vi "initialise.vi"(8 "error in (no error)":errorcluster, 11 "GenericPlugin in":refnum<class "StageMMS2015ASIfromScientifica.lvclass">) -> (0 "error out":errorcluster, 3 "GenericPlugin out":refnum<class "StageMMS2015ASIfromScientifica.lvclass">)   [LabVIEW 2010, in "StageMMS2015ASIfromScientifica.lvclass"]
doc: "The dynamic dispatch-version of this VI initalises the plug-in object by allocating and initalising any dynamic resources need."
uses:
  StageMMS2015ASIfromScientifica.lvclass
  StageDL090409Scaffold/StageDL090409Scaffold/StageDL090409Scaffold.lvclass
  <vilib>/Instr/_visa.llb/VISA Configure Serial Port (Instr).vi
  common/classes/ErrorController/ErrorController/class_data.vi
  common/classes/ErrorController/ErrorController/ErrorController.lvclass
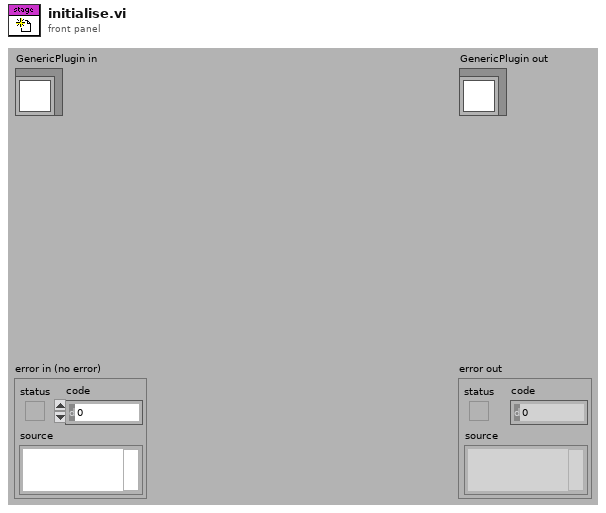
[diagram p1: front panel]
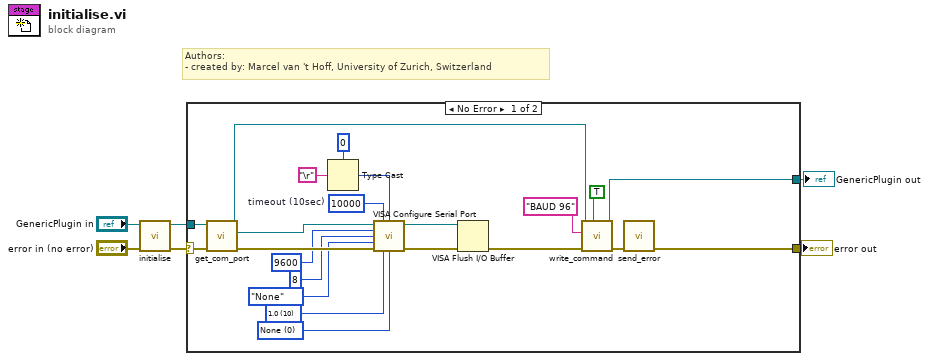
[diagram p0: block diagram]
diagram:
  # "Authors: \n- created by: Marcel van 't Hoff, University of Zurich, Switzerland"
  n1 = call-parent "initialise.vi"("error in (no error)"="error in (no error)", "GenericPlugin in"="GenericPlugin in") -> ("error out"=w4:errorcluster, "GenericPlugin out"=w1:refnum<class "StageMMS2015ASIfromScientifica.lvclass">)  [unwired: 8 in]
  n2 = case shown="No Error" w4 {
    selector: w4 -> [w26 w30]
    tunnel: [w14 w30] -> w3
    tunnel: [w17 w29] -> w2
    tunnel: w1 -> [w28 w29]
    frame No Error {
      w19 = u16 0 items=["None", "XON/XOFF", "RTS/CTS", "XON/XOFF & RTS/CTS", "DTR/DSR", "XON/XOFF & DTR/DSR"] ("flow control (0:none)")
      w20 = u16 10 items=["1.0"=10, "1.5"=15, "2.0"=20] ("stop bits (10: 1 bit)")
      w24 = u32 10000  # timeout (10sec)
      n3 = call-dynamic "get_com_port.vi"("error in (no error)"=w26, "StageMH110930Scientifica in"=w28) -> ("error out"=w25:errorcluster, "serial port name"=w27:refnum<visa-resource-name>, "StageMH110930Scientifica out"=w18:refnum<class "StageMMS2015ASIfromScientifica.lvclass">)  [unwired: 7 in]
      n4 = Type Cast(type=u8 0, x="\r") -> (*(type *) &x=w8:u8)
      n5 = call-poly "VISA Configure Serial Port"("VISA resource name"=w27, "timeout (10sec)"=w24, "termination char\n(0xA = '\\n' = LF)"=w8, "baud rate (9600)"=u32 9600, "data bits (8)"=u16 8, "parity (0:none)"=enum16{"None", "Odd", "Even", "Mark", "Space"}."None", "error in (no error)"=w25, "stop bits (10: 1 bit)"=w20, "flow control (0:none)"=w19) -> ("VISA resource name out"=w12:refnum<visa-resource-name>, "error out"=w11:errorcluster)  [unwired: 5 in]
      n6 = VISA Flush I/O Buffer(VISA resource name=w12, error in (no error)=w11) -> (error out=w10:errorcluster)  [unwired: 1 in, 1 out]
      n7 = call-dynamic "write_command.vi"("read (T)"=TRUE, "error in (no error)"=w10, "string to write"="BAUD 96", "StageMH110930Scientifica in"=w18) -> ("error out"=w15:errorcluster, "StageMH110930Scientifica out"=w17:refnum<class "StageMMS2015ASIfromScientifica.lvclass">)  [unwired: 4 in, 2 out]
      n8 = call "send_error.vi"("error in (no error)"=w15) -> ("error out"=w14:errorcluster)  [unwired: 10 in]
    }
    frame Error {
    }
  }
  "error out" <- w3
  "GenericPlugin out" <- w2
